vi "Deq Host Data (SubVI).vi"(7 "Host Data":string, 8 "error in (no error)":errorcluster) -> (0 "error out":errorcluster, 1 "Data Out":string[](array[string]), 2 "CPU out":T1, 3 "output Data":T2, 5 "IP out":string)   [LabVIEW 2021]
uses:
  Main Engine/Controls/Main Engine CPU Info.ctl
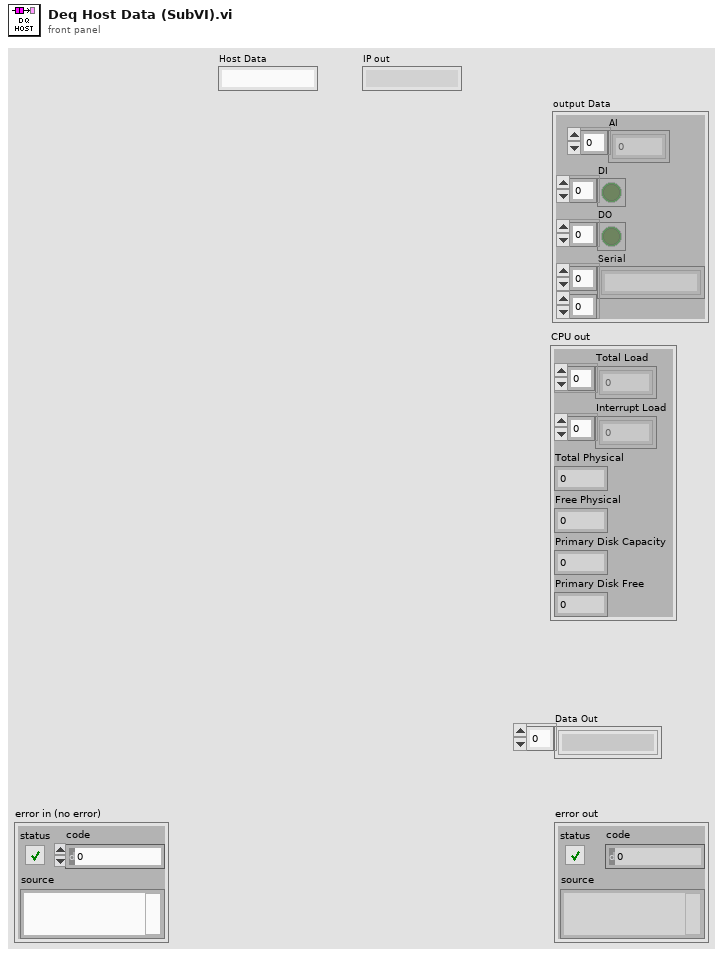
[diagram p1: front panel]
types:
  T1 = typedef "Main Engine CPU Info.ctl" = cluster{"Total Load":u32[], "Interrupt Load":u32[], "Total Physical":dbl, "Free Physical":dbl, "Primary Disk Capacity":dbl, "Primary Disk Free":dbl}
  T2 = cluster{"AI":dbl[], "DI":bool[], "DO":bool[], "Serial":string[][]}
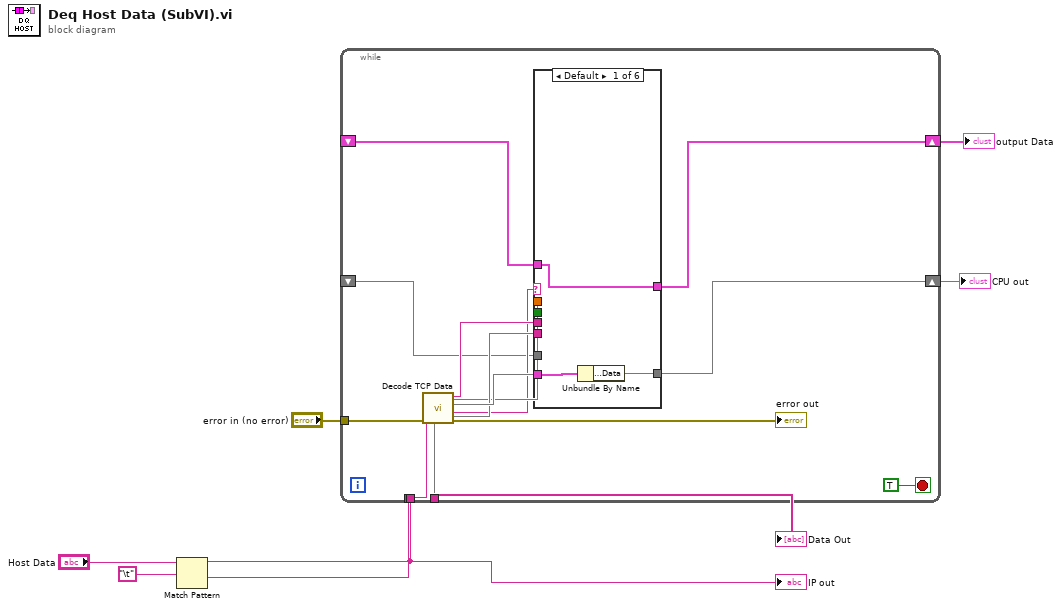
[diagram p0: block diagram]
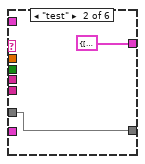
[diagram p2: hidden frame]
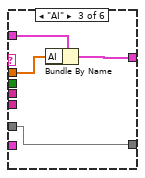
[diagram p3: hidden frame]
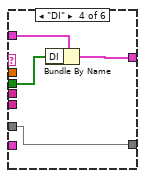
[diagram p4: hidden frame]
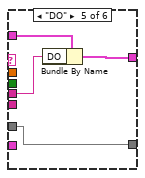
[diagram p5: hidden frame]
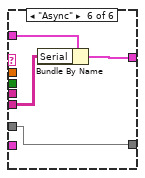
[diagram p6: hidden frame]
diagram:
  n1 = Match Pattern(string="Host Data", regular expression="\t") -> (before substring=w4:string, after substring=w5:string)  [unwired: 1 in, 2 out]
  "IP out" <- w4
  n2 = while {
    tunnel: "error in (no error)" -> [w23]
    tunnel: [w15] -> w6
    tunnel: w5 -> [w14]
    tunnel: w4 -> [_]
    shift-right: [w13] -> w1
    shift-left: _ -> [w12]
    shift-right: [w9] -> w2
    shift-left: _ -> [w10]
    stop <- TRUE stop-if-true
    n3 = call "Decode TCP Data.vi"("error in"=w23, 11:w14) -> ("error out"=→"error out":errorcluster, "Type"=w16:string, 2:w21, "Input Data out"=w19:string, 4:w20, 5:w18, 6:w15, 7:w17)  [unwired: 2 in]
    n4 = case shown="Default" w16 {
      tunnel: w12 -> [w26 _ w32 w36 w40 w44]
      tunnel: w17 -> [_ _ w31 _ _ _]
      tunnel: w18 -> [_ _ _ w34 _ _]
      tunnel: w19 -> [_ _ _ _ w38 _]
      tunnel: w20 -> [_ _ _ _ _ w42]
      tunnel: [w26 T2 {"AI"=[], "DI"=[], "DO"=[], "Serial"=[]} ("output Data") w30 w35 w39 w43] -> w13
      tunnel: w21 -> [w25 _ _ _ _ _]
      tunnel: [w24 w28 w29 w33 w37 w41] -> w9
      tunnel: w10 -> [_ w28 w29 w33 w37 w41]
      frame Default {
        n5 = Unbundle By Name(w25) -> ("Interface Data.Data"=w24)
      }
      frame "test" {
      }
      frame "AI" {
        n6 = Bundle By Name(cluster=w32, "AI"=w31) -> (w30:T2)
      }
      frame "DI" {
        n7 = Bundle By Name(cluster=w36, "DI"=w34) -> (w35:T2)
      }
      frame "DO" {
        n8 = Bundle By Name(cluster=w40, "DO"=w38) -> (w39:T2)
      }
      frame "Async" {
        n9 = Bundle By Name(cluster=w44, "Serial"=w42) -> (w43:T2)
      }
    }
  }
  "Data Out" <- w6
  "output Data" <- w1
  "CPU out" <- w2
